vi "LUT Tester.vi"() -> ()   [LabVIEW 2023]
panel:
  in  "Multiplier":dbl=100.0 format="%#_13g"
  in  "Divider":dbl=1000.0 format="%#_13g"
  in  "Power":dbl=0.5 format="%#_13g"
  out "LUT":dbl[](graph)=[-35.63705936241092, -35.49647869859769, -35.35533905932738, -35.21363372331802, -35.07135583350036, -34.928498393145965, -34.785054261852174, -34.64101615137755, -34.49637662132068, -34.351128074635334, -34.20526275297414, -34.058772731852805, -33.91164991562634, -33.76388603226827, -33.61547262794322, -33.46640106136302, -33.31666249791536, -33.166247903553995, -33.015148038438355, -32.863353450309965, -32.710854467592256, -32.55764119219941, -32.4037034920393, -32.2490309931942, -32.09361307176242, -31.937438845342626, -31.78049716414141, -31.622776601683793, -31.464265445104544, -31.304951684997057, -31.144823004794876, -30.983866769659336, -30.822070014844883, -30.65941943351178, -30.495901363953813, -30.331501776206203, -30.166206257996713, -30.0, -29.832867780352597, -29.664793948382652, -29.49576240750525, -29.325756597230356, -29.154759474226505, -28.982753492378876, -28.809720581775867, -28.635642126552707, -28.460498941515418, -28.284271247461902, -28.10693864511039, -27.92848008753788, -27.748873851023216, -27.568097504180443, -27.386127875258303, -27.202941017470888, -27.01851217221259, -26.832815729997478, -26.645825188948454, -26.45751311064591, -26.267851073127396, -26.076809620810597, -25.88435821108957, -25.690465157330262, -25.495097567963924, -25.298221281347033, -25.099800796022265, -24.899799195977465, -24.69817807045694, -24.49489742783178, -24.289915602982237, -24.08318915758459, -23.874672772626646, -23.664319132398465, -23.45207879911715, -23.2379000772445, -23.021728866442675, -22.80350850198276, -22.58317958127243, -22.360679774997898, -22.135943621178654, -21.908902300206645, -21.6794833886788, -21.447610589527216, -21.213203435596427, -20.97617696340303, -20.73644135332772, -20.4939015319192, -20.248456731316587, -20.0, -19.748417658131498, -19.493588689617926, -19.235384061671347, -18.973665961010276, -18.708286933869708, -18.439088914585774, -18.16590212458495, -17.88854381999832, -17.60681686165901, -17.320508075688775, -17.029386365926403, -16.73320053068151, -16.431676725154983, -16.1245154965971, -15.811388300841896, -15.491933384829668, -15.165750888103101, -14.832396974191326, -14.491376746189438, -14.142135623730951, -13.784048752090222, -13.416407864998739, -13.038404810405298, -12.649110640673516, -12.24744871391589, -11.832159566199232, -11.40175425099138, -10.954451150103322, -10.488088481701515, -10.0, -9.486832980505138, -8.94427190999916, -8.366600265340756, -7.745966692414834, -7.0710678118654755, -6.324555320336758, -5.477225575051661, -4.47213595499958, -3.162277660168379, 0.0, 3.162277660168379, 4.47213595499958, 5.477225575051661, 6.324555320336758, 7.0710678118654755, 7.745966692414834, 8.366600265340756, 8.94427190999916, 9.486832980505138, 10.0, 10.488088481701515, 10.954451150103322, 11.40175425099138, 11.832159566199232, 12.24744871391589, 12.649110640673516, 13.038404810405298, 13.416407864998739, 13.784048752090222, 14.142135623730951, 14.491376746189438, 14.832396974191326, 15.165750888103101, 15.491933384829668, 15.811388300841896, 16.1245154965971, 16.431676725154983, 16.73320053068151, 17.029386365926403, 17.320508075688775, 17.60681686165901, 17.88854381999832, 18.16590212458495, 18.439088914585774, 18.708286933869708, 18.973665961010276, 19.235384061671347, 19.493588689617926, 19.748417658131498, 20.0, 20.248456731316587, 20.4939015319192, 20.73644135332772, 20.97617696340303, 21.213203435596427, 21.447610589527216, 21.6794833886788, 21.908902300206645, 22.135943621178654, 22.360679774997898, 22.58317958127243, 22.80350850198276, 23.021728866442675, 23.2379000772445, 23.45207879911715, 23.664319132398465, 23.874672772626646, 24.08318915758459, 24.289915602982237, 24.49489742783178, 24.69817807045694, 24.899799195977465, 25.099800796022265, 25.298221281347033, 25.495097567963924, 25.690465157330262, 25.88435821108957, 26.076809620810597, 26.267851073127396, 26.45751311064591, 26.645825188948454, 26.832815729997478, 27.01851217221259, 27.202941017470888, 27.386127875258303, 27.568097504180443, 27.748873851023216, 27.92848008753788, 28.10693864511039, 28.284271247461902, 28.460498941515418, 28.635642126552707, 28.809720581775867, 28.982753492378876, 29.154759474226505, 29.325756597230356, 29.49576240750525, 29.664793948382652, 29.832867780352597, 30.0, 30.166206257996713, 30.331501776206203, 30.495901363953813, 30.65941943351178, 30.822070014844883, 30.983866769659336, 31.144823004794876, 31.304951684997057, 31.464265445104544, 31.622776601683793, 31.78049716414141, 31.937438845342626, 32.09361307176242, 32.2490309931942, 32.4037034920393, 32.55764119219941, 32.710854467592256, 32.863353450309965, 33.015148038438355, 33.166247903553995, 33.31666249791536, 33.46640106136302, 33.61547262794322, 33.76388603226827, 33.91164991562634, 34.058772731852805, 34.20526275297414, 34.351128074635334, 34.49637662132068, 34.64101615137755, 34.785054261852174, 34.928498393145965, 35.07135583350036, 35.21363372331802, 35.35533905932738, 35.49647869859769, 35.63705936241092, 35.77708763999664]
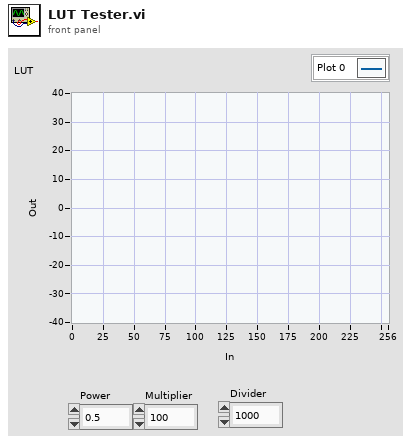
[diagram p1: front panel]
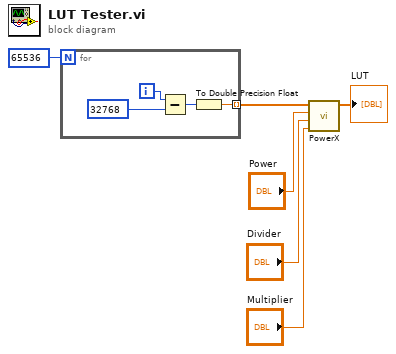
[diagram p0: block diagram]
diagram:
  n1 = for {
    N: 65536 -> [_]
    tunnel: [w10] -> w4 mode=indexing
    i -> [w9]
    n2 = Subtract(x=w9, y=32768) -> (x-y=w8:i32)
    n3 = To Double Precision Float(number=w8) -> (double precision float=w10:dbl)
  }
  n4 = call "PowerX.vi"("Multiplier"="Multiplier", "Divider"="Divider", "Power"="Power", "Signal In"=w4) -> ("Signal Out"=→"LUT":dbl[])  [unwired: 7 in]
